vi "lib path.vi"(1 "Overwrite Lib Path":path) -> (0 "lib path":path)   [LabVIEW 2020, in "KD Tree.lvlib"]
uses:
  KD Tree.lvlib
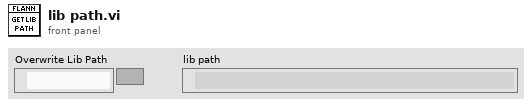
[diagram p1: front panel]
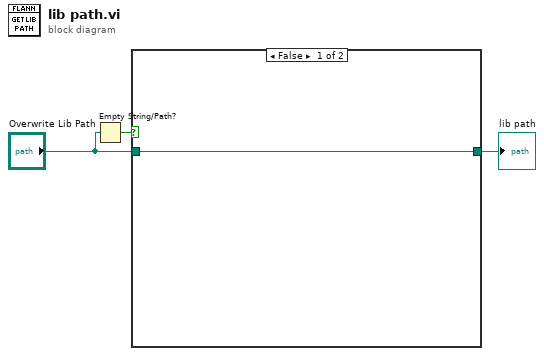
[diagram p0: block diagram]
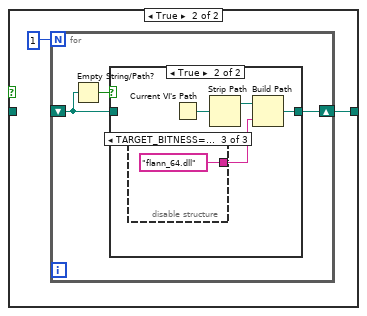
[diagram p2: hidden frame]
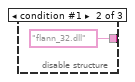
[diagram p5: hidden frame]
diagram:
  n1 = Empty String/Path?(string/path="Overwrite Lib Path") -> (empty?=w2:bool)
  n2 = case shown="False" w2 {
    tunnel: [w4 w6] -> w3
    tunnel: "Overwrite Lib Path" -> [w4 _]
    frame False {
    }
    frame True {
      n3 = for {
        N: 1 -> [_]
        shift-right: [w9] -> w6
        shift-left: _ -> [w7]
        n4 = Empty String/Path?(string/path=w7) -> (empty?=w8:bool)
        n5 = case shown="True" w8 {
          tunnel: [w10 w14] -> w9
          tunnel: w7 -> [w10 _]
          frame False {
          }
          frame True {
            n6 = disable-structure shown="TARGET_BITNESS==64" {
              disable-tunnel: [_ "flann_32.dll" "flann_64.dll"] -> w11
              frame condition #0 {
              }
              frame condition #1 {
              }
              frame condition #2 (active) {
              }
            }
            n7 = Current VI's Path() -> (path=w13:path)
            n8 = Strip Path(path=w13) -> (stripped path=w12:path)  [unwired: 1 out]
            n9 = Build Path(base path=w12, name or relative path=w11) -> (appended path=w14:path)
          }
        }
      }
    }
  }
  "lib path" <- w3
